vi "rszvl_core_global.vi"() -> ()   [LabVIEW 2014] (continued)
Low,Upp\r\n\nRemote-control command(s):\nCALCulate<1|2>:ATV:LIMit:RESult:CARRiers:<S1PRelative | S2PRelative>:<LOWer | UPPer>?", "Flags"={"OPC Wait"=FALSE, "Dont check status"=FALSE, "*WAI"=FALSE}, "Check Status Callback"=""}, {"Level"=3, "Descriptive Name"="CATV Analog TV Frequency Offset Limit, Vision Carrier Result", "Class Only"=FALSE, "Data Type"=0, "Access"=0, "Identifier"="RSZVL_ATTR_CATV_ATV_CARR_LIM_VCF_RESULT", "Range Table"="rszvl_rngCatvResults", "Command"="CALC:ATV:LIM:RES:CARR:VCF:{ModifLowUpp}?", "Read Callback"="", "Write Callback"="", "Range Callback"="", "Check Callback"="", "Rngtable Callback"="", "Coerce Callback"="", "User Callback"="", "Supported Models"="", "Instrument Options"="", "Repeated Capabilities"="", "Restricted Repeated Capabilities"="", "Help"="This attribute performs a limit check for the frequency offset of the vision carrier.\n\nAvailable Repeated Capabilities:\nModifLowUpp: Low,Upp\r\n\nRemote-control command(s):\nCALCulate<1|2>:ATV:LIMit:RESult:CARRiers:VCFoffset:<LOWer | UPPer>?", "Flags"={"OPC Wait"=FALSE, "Dont check status"=FALSE, "*WAI"=FALSE}, "Check Status Callback"=""}, {"Level"=3, "Descriptive Name"="CATV Analog TV Absolute Limit, Vision Carrier Result", "Class Only"=FALSE, "Data Type"=0, "Access"=0, "Identifier"="RSZVL_ATTR_CATV_ATV_CARR_LIM_VCP_RESULT", "Range Table"="rszvl_rngCatvResults", "Command"="CALC:ATV:LIM:RES:CARR:VCP:{ModifLowUpp}?", "Read Callback"="", "Write Callback"="", "Range Callback"="", "Check Callback"="", "Rngtable Callback"="", "Coerce Callback"="", "User Callback"="", "Supported Models"="", "Instrument Options"="", "Repeated Capabilities"="", "Restricted Repeated Capabilities"="", "Help"="This attribute performs a limit check for the absolute vision carrier power.\n\nAvailable Repeated Capabilities:\nModifLowUpp: Low,Upp\r\n\nRemote-control command(s):\nCALCulate<1|2>:ATV:LIMit:RESult:CARRiers:VCPabsolute:<LOWer | UPPer>?", "Flags"={"OPC Wait"=FALSE, "Dont check status"=FALSE, "*WAI"=FALSE}, "Check Status Callback"=""}, {"Level"=3, "Descriptive Name"="CATV Analog TV Carrier to Noise Ratio Limit Result", "Class Only"=FALSE, "Data Type"=0, "Access"=0, "Identifier"="RSZVL_ATTR_CATV_ATV_LIM_CN_RESULT", "Range Table"="rszvl_rngCatvResults", "Command"="CALC:ATV:LIM:RES:CN:CN:{ModifLowUpp}?", "Read Callback"="", "Write Callback"="", "Range Callback"="", "Check Callback"="", "Rngtable Callback"="", "Coerce Callback"="", "User Callback"="", "Supported Models"="", "Instrument Options"="", "Repeated Capabilities"="", "Restricted Repeated Capabilities"="", "Help"="This attribute performs a limit check for the carrier–to–noise ratio.\n\nNote:\n\n(1) Only Lower Limit is available.\n\nAvailable Repeated Capabilities:\nModifLowUpp: Low,Upp\r\n\nRemote-control command(s):\nCALCulate<1|2>:ATV:LIMit:RESult:CN:CN[:LOWer]?", "Flags"={"OPC Wait"=FALSE, "Dont check status"=FALSE, "*WAI"=FALSE}, "Check Status Callback"=""}, {"Level"=3, "Descriptive Name"="CATV Analog TV Carrier to Second Order Beat Ratio Limit Result", "Class Only"=FALSE, "Data Type"=0, "Access"=0, "Identifier"="RSZVL_ATTR_CATV_ATV_LIM_CSO_RESULT", "Range Table"="rszvl_rngCatvResults", "Command"="CALC:ATV:LIM:RES:CSO:CSO:{ModifLowUpp}?", "Read Callback"="", "Write Callback"="", "Range Callback"="", "Check Callback"="", "Rngtable Callback"="", "Coerce Callback"="", "User Callback"="", "Supported Models"="", "Instrument Options"="", "Repeated Capabilities"="", "Restricted Repeated Capabilities"="", "Help"="This attribute performs a limit check for the carrier–to–second order beat ratio.\n\nNote:\n\n(1) Only Lower Limit is available\n\nAvailable Repeated Capabilities:\nModifLowUpp: Low,Upp\r\n\nRemote-control command(s):\nCALCulate<1|2>:ATV:LIMit:RESult:CSO:CSO[:LOWer]?", "Flags"={"OPC Wait"=FALSE, "Dont check status"=FALSE, "*WAI"=FALSE}, "Check Status Callback"=""}, {"Level"=3, "Descriptive Name"="CATV Analog TV Carrier to Composite Triple Beat Ratio Limit Result", "Class Only"=FALSE, "Data Type"=0, "Access"=0, "Identifier"="RSZVL_ATTR_CATV_ATV_LIM_CTB_RESULT", "Range Table"="rszvl_rngCatvResults", "Command"="CALC:ATV:LIM:RES:CTB:CTB:{ModifLowUpp}?", "Read Callback"="", "Write Callback"="", "Range Callback"="", "Check Callback"="", "Rngtable Callback"="", "Coerce Callback"="", "User Callback"="", "Supported Models"="", "Instrument Options"="", "Repeated Capabilities"="", "Restricted Repeated Capabilities"="", "Help"="This attribute performs a limit check for the carrier–to–composite triple beat ratio.\n\nNote:\n\n(1) Only Lower Limit is available.\n\nAvailable Repeated Capabilities:\nModifLowUpp: Low,Upp\r\n\nRemote-control command(s):\nCALCulate<1|2>:ATV:LIMit:RESult:CTB:CTB[:LOWer]?", "Flags"={"OPC Wait"=FALSE, "Dont check status"=FALSE, "*WAI"=FALSE}, "Check Status Callback"=""}, {"Level"=3, "Descriptive Name"="CATV Analog TV Hum Limit Result", "Class Only"=FALSE, "Data Type"=0, "Access"=0, "Identifier"="RSZVL_ATTR_CATV_ATV_LIM_HUM_RESULT", "Range Table"="rszvl_rngCatvResults", "Command"="CALC:ATV:LIM:RES:HUM:HUM:{ModifLowUpp}?", "Read Callback"="", "Write Callback"="", "Range Callback"="", "Check Callback"="", "Rngtable Callback"="", "Coerce Callback"="", "User Callback"="", "Supported Models"="", "Instrument Options"="", "Repeated Capabilities"="", "Restricted Repeated Capabilities"="", "Help"="This attribute performs a limit check for the Hum measurement.\n\nAvailable Repeated Capabilities:\nModifLowUpp: Low,Upp\r\n\nRemote-control command(s):\nCALCulate<1|2>:ATV:LIMit:RESult:HUM:HUM:<LOWer | UPPer>?", "Flags"={"OPC Wait"=FALSE, "Dont check status"=FALSE, "*WAI"=FALSE}, "Check Status Callback"=""}, {"Level"=3, "Descriptive Name"="CATV Analog TV Vision Modulation Result", "Class Only"=FALSE, "Data Type"=0, "Access"=0, "Identifier"="RSZVL_ATTR_CATV_ATV_LIM_VMOD_MDEP_RESULT", "Range Table"="rszvl_rngCatvResults", "Command"="CALC:ATV:LIM:RES:VMOD:{AtvVisionModulResult}:{ModifLowUpp}?", "Read Callback"="", "Write Callback"="", "Range Callback"="", "Check Callback"="", "Rngtable Callback"="", "Coerce Callback"="", "User Callback"="", "Supported Models"="", "Instrument Options"="", "Repeated Capabilities"="", "Restricted Repeated Capabilities"="", "Help"="This attribute performs a limit check for the  Vision Modulation measurement.\n\nAvailable Repeated Capabilities:\nAtvVisionModulResult: VisCarrPow,ResPicture,Depth\r\nModifLowUpp: Low,Upp\r\n\nRemote-control command(s):\nCALCulate<1|2>:ATV:LIMit:RESult:VMODulation:<MDEPth|RPC|VCP>:<LOWer | UPPer>?", "Flags"={"OPC Wait"=FALSE, "Dont check status"=FALSE, "*WAI"=FALSE}, "Check Status Callback"=""}, {"Level"=2, "Descriptive Name"="ATV Results", "Class Only"=TRUE, "Data Type"=0, "Access"=0, "Identifier"="", "Range Table"="", "Command"="", "Read Callback"="", "Write Callback"="", "Range Callback"="", "Check Callback"="", "Rngtable Callback"="", "Coerce Callback"="", "User Callback"="", "Supported Models"="", "Instrument Options"="", "Repeated Capabilities"="", "Restricted Repeated Capabilities"="", "Help"="Attributes that return ATV measurement results.\n\n(1) CATV Get Analog TV Vision Carrier Power Abs:\nThis attribute reads the vision carrier power absolute value of the Carrier Power measurements.\n\n(2) CATV Get Analog TV Vision Carrier Frequency Offset Value:\nThis attribute reads the vision carrier frequency offset value of the Carrier Power measurements.\n\n(3) CATV Get Analog TV Sound Carrier Power Rel Value:\nThis attribute reads the sound carrier power relative value of the Carrier Power measurements.\n\n(4) CATV Get Analog TV Sound Carrier Intercarrier Frequency Offset Value:\nThis attribute reads the sound carrier intercarrier frequency offset value of the Carrier Power measurements.\n\n(5) CATV Get Analog TV Carrier Result Value:\nThis attribute reads the value of the measurements.\n\nNote:\n\n(1) NRBW is valid only for CN measurement\n\n(6) CATV Get Analog TV CN Carrier to Noise Ratio Value:\nThis attribute reads the carrier–to–noise ratio value of the Carrier–to–Noise Ratio measurements.\n\n(7) CATV Get Analog TV CSO Carrier to Second Order Beat Ratio Value:\nThis attribute reads the carrier–to–second order beat ratio value of the Carrier–to–Second Order Beat Ratio measurements.\n\n(8) CATV Get Analog TV CTB Carrier to Composite Triple Beat Ratio Value:\nThis attribute reads the carrier–to–to–composite triple beat beat ratio value of the Carrier–to–Composite Trip Beat Ratio measurements.\n\n(9) CATV Get Analog TV Hum Value:\nThis attribute reads the measurement values of the Hum measurement.\n\n(10) CATV Get Analog TV Vision Modulation Result Value:\nThis attribute reads the result value of Vision Modulation measurements.", "Flags"={"OPC Wait"=FALSE, "Dont check status"=FALSE, "*WAI"=FALSE}, "Check Status Callback"=""}, {"Level"=3, "Descriptive Name"="CATV Get Analog TV Vision Carrier Power Abs", "Class Only"=FALSE, "Data Type"=1, "Access"=0, "Identifier"="RSZVL_ATTR_CATV_ATV_CARR_VCPA", "Range Table"="", "Command"="CALC:ATV:RES:CARR? VCP", "Read Callback"="", "Write Callback"="", "Range Callback"="", "Check Callback"="", "Rngtable Callback"="", "Coerce Callback"="", "User Callback"="", "Supported Models"="", "Instrument Options"="", "Repeated Capabilities"="", "Restricted Repeated Capabilities"="", "Help"="This attribute reads the vision carrier power absolute value of the Carrier Power measurements.\n\nAvailable Repeated Capabilities:\nNone\n\nRemote-control command(s):\nCALCulate<1|2>:ATV:RESult:CARRiers? VCPabsolute", "Flags"={"OPC Wait"=FALSE, "Dont check status"=FALSE, "*WAI"=FALSE}, "Check Status Callback"=""}, {"Level"=3, "Descriptive Name"="CATV Get Analog TV Vision Carrier Frequency Offset Value", "Class Only"=FALSE, "Data Type"=1, "Access"=0, "Identifier"="RSZVL_ATTR_CATV_ATV_CARR_VCF_VALUE", "Range Table"="", "Command"="CALC:ATV:RES:CARR? VCF", "Read Callback"="", "Write Callback"="", "Range Callback"="", "Check Callback"="", "Rngtable Callback"="", "Coerce Callback"="", "User Callback"="", "Supported Models"="", "Instrument Options"="", "Repeated Capabilities"="", "Restricted Repeated Capabilities"="", "Help"="This attribute reads the vision carrier frequency offset value of the Carrier Power measurements.\n\nAvailable Repeated Capabilities:\nNone\n\nRemote-control command(s):\nCALCulate<1|2>:ATV:RESult:CARRiers? VCFoffset", "Flags"={"OPC Wait"=FALSE, "Dont check status"=FALSE, "*WAI"=FALSE}, "Check Status Callback"=""}, {"Level"=3, "Descriptive Name"="CATV Get Analog TV Sound Carrier Power Rel Value", "Class Only"=FALSE, "Data Type"=1, "Access"=0, "Identifier"="RSZVL_ATTR_CATV_ATV_CARR_REL_POWER_VALUE", "Range Table"="", "Command"="CALC:ATV:RES:CARR? {AtvSoundCarrier}PR", "Read Callback"="", "Write Callback"="", "Range Callback"="", "Check Callback"="", "Rngtable Callback"="", "Coerce Callback"="", "User Callback"="", "Supported Models"="", "Instrument Options"="", "Repeated Capabilities"="", "Restricted Repeated Capabilities"="", "Help"="This attribute reads the sound carrier power relative value of the Carrier Power measurements.\n\nAvailable Repeated Capabilities:\nAtvSoundCarrier: SC1,SC2\r\n\nRemote-control command(s):\nCALCulate<1|2>:ATV:RESult:CARRiers? S1PRelative | S2PRelative", "Flags"={"OPC Wait"=FALSE, "Dont check status"=FALSE, "*WAI"=FALSE}, "Check Status Callback"=""}, {"Level"=3, "Descriptive Name"="CATV Get Analog TV Sound Carrier Intercarrier Frequency Offset Value", "Class Only"=FALSE, "Data Type"=1, "Access"=0, "Identifier"="RSZVL_ATTR_CATV_ATV_CARR_FREQ_OFFSET_VALUE", "Range Table"="", "Command"="CALC:ATV:RES:CARR? {AtvSoundCarrier}IF", "Read Callback"="", "Write Callback"="", "Range Callback"="", "Check Callback"="", "Rngtable Callback"="", "Coerce Callback"="", "User Callback"="", "Supported Models"="", "Instrument Options"="", "Repeated Capabilities"="", "Restricted Repeated Capabilities"="", "Help"="This attribute reads the sound carrier intercarrier frequency offset value of the Carrier Power measurements.\n\nAvailable Repeated Capabilities:\nAtvSoundCarrier: SC1,SC2\r\n\nRemote-control command(s):\nCALCulate<1|2>:ATV:RESult:CARRiers? S1IFoffset | S2IFoffset", "Flags"={"OPC Wait"=FALSE, "Dont check status"=FALSE, "*WAI"=FALSE}, "Check Status Callback"=""}, {"Level"=3, "Descriptive Name"="CATV Get Analog TV Carrier Result Value", "Class Only"=FALSE, "Data Type"=1, "Access"=0, "Identifier"="RSZVL_ATTR_CATV_ATV_VALUE", "Range Table"="", "Command"="CALC:ATV:RES:{AtvCarrier}? {AtvCarrierResult}", "Read Callback"="", "Write Callback"="", "Range Callback"="", "Check Callback"="", "Rngtable Callback"="", "Coerce Callback"="", "User Callback"="", "Supported Models"="", "Instrument Options"="", "Repeated Capabilities"="", "Restricted Repeated Capabilities"="", "Help"="This attribute reads the value of the measurements.\n\nNote:\n\n(1) NRBW is valid only for CN measurement\n\nAvailable Repeated Capabilities:\nAtvCarrier: CN,CSO,CTB\r\nAtvCarrierResult: RefPow,NoiseFloorCorr,FreqRel,CR,NoiseRefBw\r\n\nRemote-control command(s):\nCALCulate<1|2>:ATV:RESult:<CN | CSO | CTB>? RPOWer | NFC | MFR | NRBW", "Flags"={"OPC Wait"=FALSE, "Dont check status"=FALSE, "*WAI"=FALSE}, "Check Status Callback"=""}, {"Level"=3, "Descriptive Name"="CATV Get Analog TV CN Carrier to Noise Ratio Value", "Class Only"=FALSE, "Data Type"=1, "Access"=0, "Identifier"="RSZVL_ATTR_CATV_ATV_CN_CN_VALUE", "Range Table"="", "Command"="CALC:ATV:RES:CN? CN", "Read Callback"="", "Write Callback"="", "Range Callback"="", "Check Callback"="", "Rngtable Callback"="", "Coerce Callback"="", "User Callback"="", "Supported Models"="", "Instrument Options"="", "Repeated Capabilities"="", "Restricted Repeated Capabilities"="", "Help"="This attribute reads the carrier–to–noise ratio value of the Carrier–to–Noise Ratio measurements.\n\nAvailable Repeated Capabilities:\nNone\n\nRemote-control command(s):\nCALCulate<1|2>:ATV:RESult:CN? CN", "Flags"={"OPC Wait"=FALSE, "Dont check status"=FALSE, "*WAI"=FALSE}, "Check Status Callback"=""}, {"Level"=3, "Descriptive Name"="CATV Get Analog TV CSO Carrier to Second Order Beat Ratio Value", "Class Only"=FALSE, "Data Type"=1, "Access"=0, "Identifier"="RSZVL_ATTR_CATV_ATV_CSO_CSO_VALUE", "Range Table"="", "Command"="CALC:ATV:RES:CSO? CSO", "Read Callback"="", "Write Callback"="", "Range Callback"="", "Check Callback"="", "Rngtable Callback"="", "Coerce Callback"="", "User Callback"="", "Supported Models"="", "Instrument Options"="", "Repeated Capabilities"="", "Restricted Repeated Capabilities"="", "Help"="This attribute reads the carrier–to–second order beat ratio value of the Carrier–to–Second Order Beat Ratio measurements.\n\nAvailable Repeated Capabilities:\nNone\n\nRemote-control command(s):\nCALCulate<1|2>:ATV:RESult:CSO? CSO", "Flags"={"OPC Wait"=FALSE, "Dont check status"=FALSE, "*WAI"=FALSE}, "Check Status Callback"=""}, {"Level"=3, "Descriptive Name"="CATV Get Analog TV CTB Carrier to Composite Triple Beat Ratio Value", "Class Only"=FALSE, "Data Type"=1, "Access"=0, "Identifier"="RSZVL_ATTR_CATV_ATV_CTB_CTB_VALUE", "Range Table"="", "Command"="CALC:ATV:RES:CTB? CTB", "Read Callback"="", "Write Callback"="", "Range Callback"="", "Check Callback"="", "Rngtable Callback"="", "Coerce Callback"="", "User Callback"="", "Supported Models"="", "Instrument Options"="", "Repeated Capabilities"="", "Restricted Repeated Capabilities"="", "Help"="This attribute reads the carrier–to–to–composite triple beat beat ratio value of the Carrier–to–Composite Trip Beat Ratio measurements.\n\nAvailable Repeated Capabilities:\nNone\n\nRemote-control command(s):\nCALCulate<1|2>:ATV:RESult:CTB? CTB", "Flags"={"OPC Wait"=FALSE, "Dont check status"=FALSE, "*WAI"=FALSE}, "Check Status Callback"=""}, {"Level"=3, "Descriptive Name"="CATV Get Analog TV Hum Value", "Class Only"=FALSE, "Data Type"=1, "Access"=0, "Identifier"="RSZVL_ATTR_CATV_ATV_HUM_VALUE", "Range Table"="", "Command"="CALC:ATV:RES:HUM?", "Read Callback"="", "Write Callback"="", "Range Callback"="", "Check Callback"="", "Rngtable Callback"="", "Coerce Callback"="", "User Callback"="", "Supported Models"="", "Instrument Options"="", "Repeated Capabilities"="", "Restricted Repeated Capabilities"="", "Help"="This attribute reads the measurement values of the Hum measurement.\n\nAvailable Repeated Capabilities:\nNone\n\nRemote-control command(s):\nCALCulate<1|2>:ATV:RESult:HUM?", "Flags"={"OPC Wait"=FALSE, "Dont check status"=FALSE, "*WAI"=FALSE}, "Check Status Callback"=""}, {"Level"=3, "Descriptive Name"="CATV Get Analog TV Vision Modulation Result Value", "Class Only"=FALSE, "Data Type"=1, "Access"=0, "Identifier"="RSZVL_ATTR_CATV_ATV_VMOD_RESULT_VALUE", "Range Table"="", "Command"="CALC:ATV:RES:VMOD? {AtvVisionModulResult}", "Read Callback"="", "Write Callback"="", "Range Callback"="", "Check Callback"="", "Rngtable Callback"="", "Coerce Callback"="", "User Callback"="", "Supported Models"="", "Instrument Options"="", "Repeated Capabilities"="", "Restricted Repeated Capabilities"="", "Help"="This attribute reads the result value of Vision Modulation measurements.\n\nAvailable Repeated Capabilities:\nAtvVisionModulResult: VisCarrPow,ResPicture,Depth\r\n\nRemote-control command(s):\nCALCulate<1|2>:ATV:RESult:VMODulation? VCPower | RPC | MDEPth", "Flags"={"OPC Wait"=FALSE, "Dont check status"=FALSE, "*WAI"=FALSE}, "Check Status Callback"=""}, {"Level"=2, "Descriptive Name"="DTV Settings", "Class Only"=TRUE, "Data Type"=0, "Access"=0, "Identifier"="", "Range Table"="", "Command"="", "Read Callback"="", "Write Callback"="", "Range Callback"="", "Check Callback"="", "Rngtable Callback"="", "Coerce Callback"="", "User Callback"="", "Supported Models"="", "Instrument Options"="", "Repeated Capabilities"="", "Restricted Repeated Capabilities"="", "Help"="Attributes that configure DTV Settings.\n\n(1) CATV Digital TV Measurement:\nThis attribute defines the digital measurement type.\n\n(2) CATV Digital TV Shoulder Measurement:\nThis attribute activates or deactivates the shoulder measurement in accordance to ETSI TR 101290 standard.\n\n(3) CATV Digital TV Echo Pattern Units:\nThis attribute defines the unit of the Echo Pattern measurement.\n\n(4) CATV Digital TV Echo Pattern Velocity Factor:\nThis attribute defines the velocity of propagation of the signal in the transmission channel (e.g. cable), relative to speed of light.\n\n(5) CATV Digital TV Error Measurements Units:\nThis attribute defines the unit in the Overview / Modulation Errors measurement.\n\n(6) CATV Digital TV Equalizer State:\nThis attribute activates or deactivates the equalizer.\n\n(7) CATV Digital TV Equalizer Freeze:\nThis attribute defines the change of the equalizer coefficients.\n\n(8) CATV Digital TV Equalizer Reset:\nThis attribute resets the equalizer and all equalizer parameters are set to their default values.\n\n(9) CATV Digital TV Roll Off:\nThis attribute defines the roll–off.\n\n(10) CATV Digital TV Symbol Rate:\nThis attribute defines the symbol rate.\n\n(11) CATV Digital TV Standard:\nThis attribute sets the TV standard for Digital TV\n\n(12) CATV Digital TV Constellation Parameter:\nThis attribute sets the constellation parameter for digital TV measurements.", "Flags"={"OPC Wait"=FALSE, "Dont check status"=FALSE, "*WAI"=FALSE}, "Check Status Callback"=""}, {"Level"=3, "Descriptive Name"="CATV Digital TV Measurement", "Class Only"=FALSE, "Data Type"=0, "Access"=2, "Identifier"="RSZVL_ATTR_CATV_DTV_MEAS", "Range Table"="rszvl_rngCatvDtvMeas", "Command"="CONF:DTV:MEAS", "Read Callback"="", "Write Callback"="", "Range Callback"="", "Check Callback"="", "Rngtable Callback"="", "Coerce Callback"="", "User Callback"="", "Supported Models"="", "Instrument Options"="", "Repeated Capabilities"="", "Restricted Repeated Capabilities"="", "Help"="This attribute defines the digital measurement type.\n\nAvailable Repeated Capabilities:\nNone\n\nRemote-control command(s):\nCONFigure:DTV:MEASurement DSPectrum | CHPower | CONS | MERRors | EPATtern | APD | CCDF | OVERview", "Flags"={"OPC Wait"=FALSE, "Dont check status"=FALSE, "*WAI"=FALSE}, "Check Status Callback"=""}, {"Level"=3, "Descriptive Name"="CATV Digital TV Shoulder Measurement", "Class Only"=FALSE, "Data Type"=3, "Access"=2, "Identifier"="RSZVL_ATTR_CATV_DTV_SATT", "Range Table"="", "Command"="CONF:DTV:MEAS:SATT", "Read Callback"="", "Write Callback"="", "Range Callback"="", "Check Callback"="", "Rngtable Callback"="", "Coerce Callback"="", "User Callback"="", "Supported Models"="", "Instrument Options"="", "Repeated Capabilities"="", "Restricted Repeated Capabilities"="", "Help"="This attribute activates or deactivates the shoulder measurement in accordance to ETSI TR 101290 standard.\n\nAvailable Repeated Capabilities:\nNone\n\nRemote-control command(s):\nCONFigure:DTV:MEASurement:SATTenuation ON | OFF", "Flags"={"OPC Wait"=FALSE, "Dont check status"=FALSE, "*WAI"=FALSE}, "Check Status Callback"=""}, {"Level"=3, "Descriptive Name"="CATV Digital TV Echo Pattern Units", "Class Only"=FALSE, "Data Type"=0, "Access"=2, "Identifier"="RSZVL_ATTR_CATV_DTV_EPAT_UNIT", "Range Table"="rszvl_rngUnitSecMin", "Command"="CALC:DTV:UNIT:POW:EPAT", "Read Callback"="", "Write Callback"="", "Range Callback"="", "Check Callback"="", "Rngtable Callback"="", "Coerce Callback"="", "User Callback"="", "Supported Models"="", "Instrument Options"="", "Repeated Capabilities"="", "Restricted Repeated Capabilities"="", "Help"="This attribute defines the unit of the Echo Pattern measurement.\n\nAvailable Repeated Capabilities:\nNone\n\nRemote-control command(s):\nCALCulate<1|2>:DTV:UNIT:POWer:EPATtern", "Flags"={"OPC Wait"=FALSE, "Dont check status"=FALSE, "*WAI"=FALSE}, "Check Status Callback"=""}, {"Level"=3, "Descriptive Name"="CATV Digital TV Echo Pattern Velocity Factor", "Class Only"=FALSE, "Data Type"=1, "Access"=2, "Identifier"="RSZVL_ATTR_CATV_DTV_EPAT_RVEL", "Range Table"="rszvl_rngCatvDtvEPattVelocity", "Command"="CORR:RVEL", "Read Callback"="", "Write Callback"="", "Range Callback"="", "Check Callback"="", "Rngtable Callback"="", "Coerce Callback"="", "User Callback"="", "Supported Models"="", "Instrument Options"="", "Repeated Capabilities"="", "Restricted Repeated Capabilities"="", "Help"="This attribute defines the velocity of propagation of the signal in the transmission channel (e.g. cable), relative to speed of light.\n\nAvailable Repeated Capabilities:\nNone\n\nRemote-control command(s):\n[SENSe<1|2>:]CORRection:RVELocity", "Flags"={"OPC Wait"=FALSE, "Dont check status"=FALSE, "*WAI"=FALSE}, "Check Status Callback"=""}, {"Level"=3, "Descriptive Name"="CATV Digital TV Error Measurements Units", "Class Only"=FALSE, "Data Type"=0, "Access"=2, "Identifier"="RSZVL_ATTR_CATV_DTV_ERROR_UNIT", "Range Table"="rszvl_rngUnitDbPct", "Command"="CALC:DTV:UNIT:POW:{DtvErrorMeas}", "Read Callback"="", "Write Callback"="", "Range Callback"="", "Check Callback"="", "Rngtable Callback"="", "Coerce Callback"="", "User Callback"="", "Supported Models"="", "Instrument Options"="", "Repeated Capabilities"="", "Restricted Repeated Capabilities"="", "Help"="This attribute defines the unit in the Overview / Modulation Errors measurement.\n\nAvailable Repeated Capabilities:\nDtvErrorMeas: EVMPeak,EVMRms,MERPeak,MERRms\r\n\nRemote-control command(s):\nCALCulate<1|2>:DTV:UNIT:POWer:<EVMPeak | EVMRms | MERPeak | MERRms>", "Flags"={"OPC Wait"=FALSE, "Dont check status"=FALSE, "*WAI"=FALSE}, "Check Status Callback"=""}, {"Level"=3, "Descriptive Name"="CATV Digital TV Equalizer State", "Class Only"=FALSE, "Data Type"=3, "Access"=2, "Identifier"="RSZVL_ATTR_CATV_DTV_EQUALIZER_STATE", "Range Table"="", "Command"="DDEM:EQU", "Read Callback"="", "Write Callback"="", "Range Callback"="", "Check Callback"="", "Rngtable Callback"="", "Coerce Callback"="", "User Callback"="", "Supported Models"="", "Instrument Options"="", "Repeated Capabilities"="", "Restricted Repeated Capabilities"="", "Help"="This attribute activates or deactivates the equalizer.\n\nAvailable Repeated Capabilities:\nNone\n\nRemote-control command(s):\n[SENSe<1|2>:]DDEMod:EQUalizer[:STATe]", "Flags"={"OPC Wait"=FALSE, "Dont check status"=FALSE, "*WAI"=FALSE}, "Check Status Callback"=""}, {"Level"=3, "Descriptive Name"="CATV Digital TV Equalizer Freeze", "Class Only"=FALSE, "Data Type"=3, "Access"=2, "Identifier"="RSZVL_ATTR_CATV_DTV_EQUALIZER_FREEZE", "Range Table"="", "Command"="DDEM:EQU:FRE", "Read Callback"="", "Write Callback"="", "Range Callback"="", "Check Callback"="", "Rngtable Callback"="", "Coerce Callback"="", "User Callback"="", "Supported Models"="", "Instrument Options"="", "Repeated Capabilities"="", "Restricted Repeated Capabilities"="", "Help"="This attribute defines the change of the equalizer coefficients.\n\nAvailable Repeated Capabilities:\nNone\n\nRemote-control command(s):\n[SENSe<1|2>:]DDEMod:EQUalizer:FREeze[:STATe]", "Flags"={"OPC Wait"=FALSE, "Dont check status"=FALSE, "*WAI"=FALSE}, "Check Status Callback"=""}, {"Level"=3, "Descriptive Name"="CATV Digital TV Equalizer Reset", "Class Only"=FALSE, "Data Type"=4, "Access"=1, "Identifier"="RSZVL_ATTR_CATV_DTV_EQUALIZER_RESET", "Range Table"="", "Command"="DDEM:EQU:RES", "Read Callback"="", "Write Callback"="", "Range Callback"="", "Check Callback"="", "Rngtable Callback"="", "Coerce Callback"="", "User Callback"="", "Supported Models"="", "Instrument Options"="", "Repeated Capabilities"="", "Restricted Repeated Capabilities"="", "Help"="This attribute resets the equalizer and all equalizer parameters are set to their default values.\n\nAvailable Repeated Capabilities:\nNone\n\nRemote-control command(s):\n[SENSe<1|2>:]DDEMod:EQUalizer:RESet", "Flags"={"OPC Wait"=FALSE, "Dont check status"=FALSE, "*WAI"=FALSE}, "Check Status Callback"=""}, {"Level"=3, "Descriptive Name"="CATV Digital TV Roll Off", "Class Only"=FALSE, "Data Type"=0, "Access"=2, "Identifier"="RSZVL_ATTR_CATV_DTV_FILTER_ALPHA", "Range Table"="rszvl_rngCatvDtvFilterAlpha", "Command"="DDEM:FILT:ALPH", "Read Callback"="", "Write Callback"="", "Range Callback"="", "Check Callback"="", "Rngtable Callback"="", "Coerce Callback"="", "User Callback"="", "Supported Models"="", "Instrument Options"="", "Repeated Capabilities"="", "Restricted Repeated Capabilities"="", "Help"="This attribute defines the roll–off.\n\nAvailable Repeated Capabilities:\nNone\n\nRemote-control command(s):\n[SENSe<1|2>:]DDEMod:FILTer:ALPHa", "Flags"={"OPC Wait"=FALSE, "Dont check status"=FALSE, "*WAI"=FALSE}, "Check Status Callback"=""}, {"Level"=3, "Descriptive Name"="CATV Digital TV Symbol Rate", "Class Only"=FALSE, "Data Type"=1, "Access"=2, "Identifier"="RSZVL_ATTR_CATV_DTV_SRATE", "Range Table"="", "Command"="DDEM:SRAT", "Read Callback"="", "Write Callback"="", "Range Callback"="", "Check Callback"="", "Rngtable Callback"="", "Coerce Callback"="", "User Callback"="", "Supported Models"="", "Instrument Options"="", "Repeated Capabilities"="", "Restricted Repeated Capabilities"="", "Help"="This attribute defines the symbol rate.\n\nAvailable Repeated Capabilities:\nNone\n\nRemote-control command(s):\n[SENSe<1|2>:]DDEMod:SRATe", "Flags"={"OPC Wait"=FALSE, "Dont check status"=FALSE, "*WAI"=FALSE}, "Check Status Callback"=""}, {"Level"=3, "Descriptive Name"="CATV Digital TV Standard", "Class Only"=FALSE, "Data Type"=0, "Access"=2, "Identifier"="RSZVL_ATTR_CATV_DTV_STANDARD", "Range Table"="rszvl_rngCatvDtvStandard", "Command"="SET:TV:STAN", "Read Callback"="", "Write Callback"="", "Range Callback"="", "Check Callback"="", "Rngtable Callback"="", "Coerce Callback"="", "User Callback"="", "Supported Models"="", "Instrument Options"="", "Repeated Capabilities"="", "Restricted Repeated Capabilities"="", "Help"="This attribute sets the TV standard for Digital TV\n\nAvailable Repeated Capabilities:\nNone\n\nRemote-control command(s):\nSETup:TV:STANdard J83A | J83B | J83C", "Flags"={"OPC Wait"=FALSE, "Dont check status"=FALSE, "*WAI"=FALSE}, "Check Status Callback"=""}, {"Level"=3, "Descriptive Name"="CATV Digital TV Constellation Parameter", "Class Only"=FALSE, "Data Type"=0, "Access"=2, "Identifier"="RSZVL_ATTR_CATV_DTV_FORMAT", "Range Table"="rszvl_rngCatvDtvFormat", "Command"="SOUR:DM:FORM", "Read Callback"="", "Write Callback"="", "Range Callback"="", "Check Callback"="", "Rngtable Callback"="", "Coerce Callback"="", "User Callback"="", "Supported Models"="", "Instrument Options"="", "Repeated Capabilities"="", "Restricted Repeated Capabilities"="", "Help"="This attribute sets the constellation parameter for digital TV measurements.\n\nAvailable Repeated Capabilities:\nNone\n\nRemote-control command(s):\nSOURce:DM:FORMat QAM4 | QAM16 | QAM32 | QAM64 | QAM128 | QAM256 | QAM512 | QAM1024", "Flags"={"OPC Wait"=FALSE, "Dont check status"=FALSE, "*WAI"=FALSE}, "Check Status Callback"=""}, {"Level"=2, "Descriptive Name"="DTV Limit Settings", "Class Only"=TRUE, "Data Type"=0, "Access"=0, "Identifier"="", "Range Table"="", "Command"="", "Read Callback"="", "Write Callback"="", "Range Callback"="", "Check Callback"="", "Rngtable Callback"="", "Coerce Callback"="", "User Callback"="", "Supported Models"="", "Instrument Options"="", "Repeated Capabilities"="", "Restricted Repeated Capabilities"="", "Help"="Attributes that configure DTV Limit Settings.\n\n(1) CATV Digital TV Carrier Frequency Offset Limit:\nThis attribute defines the limit of the carrier frequency offset in the Overview measurement.\n\n(2) CATV Digital TV Channel Power Limit:\nThis attribute defines the limit for the Channel Power measurement.\n\n(3) CATV Digital TV Carrier Suppression Limit:\nThis attribute defines the limit of the carrier suppression in the Modulation Errors measurement.\n\nNote:\n\n(1) Only Lower Limit is available\n\n(4) CATV Digital TV Error Limit Lower:\nThis attribute defines the lower limit of the Overview/Modulation Errors measurement.\n\n(5) CATV Digital TV Error Limit Upper:\nThis attribute defines the upper limit of the  Overview/Modulation Errors measurement.\n\n(6) CATV Digital TV IQ Imbalance Limit:\nThis attribute defines the limit of the I/Q amplitude imbalance value in the Modulation Errors measurement.\n\n(7) CATV Digital TV Phase Jitter Limit:\nThis attribute defines the upper limit of the phase jitter (root mean square value of the phase error) in the Modulation Errors measurement.\n\nNote:\n\n(1) Only Upper Limit is availlable\n\n(8) CATV Digital TV Quadrature Error Limit:\nThis attribute defines the limit of the quadrature error in the Modulation Errors measurement.\n\n(9) CATV Digital TV Symbol Rate Offset Limit:\nThis attribute defines the limit of the symbol rate offset in the Overview measurement.", "Flags"={"OPC Wait"=FALSE, "Dont check status"=FALSE, "*WAI"=FALSE}, "Check Status Callback"=""}, {"Level"=3, "Descriptive Name"="CATV Digital TV Carrier Frequency Offset Limit", "Class Only"=FALSE, "Data Type"=1, "Access"=2, "Identifier"="RSZVL_ATTR_CATV_DTV_CARR_LIM_FREQ_OFFSET", "Range Table"="rszvl_rngCatvFreqOffset", "Command"="CALC:DTV:LIM:CFOF:{ModifLowUpp}", "Read Callback"="", "Write Callback"="", "Range Callback"="", "Check Callback"="", "Rngtable Callback"="", "Coerce Callback"="", "User Callback"="", "Supported Models"="", "Instrument Options"="", "Repeated Capabilities"="", "Restricted Repeated Capabilities"="", "Help"="This attribute defines the limit of the carrier frequency offset in the Overview measurement.\n\nAvailable Repeated Capabilities:\nModifLowUpp: Low,Upp\r\n\nRemote-control command(s):\nCALCulate:DTV:LIMit:CFOFfset:<LOWer | UPPer>", "Flags"={"OPC Wait"=FALSE, "Dont check status"=FALSE, "*WAI"=FALSE}, "Check Status Callback"=""}, {"Level"=3, "Descriptive Name"="CATV Digital TV Channel Power Limit", "Class Only"=FALSE, "Data Type"=1, "Access"=2, "Identifier"="RSZVL_ATTR_CATV_DTV_LIM_CHANNEL_POWER", "Range Table"="rszvl_rngCatvAbsPower", "Command"="CALC:DTV:LIM:CHP:{ModifLowUpp}", "Read Callback"="", "Write Callback"="", "Range Callback"="", "Check Callback"="", "Rngtable Callback"="", "Coerce Callback"="", "User Callback"="", "Supported Models"="", "Instrument Options"="", "Repeated Capabilities"="", "Restricted Repeated Capabilities"="", "Help"="This attribute defines the limit for the Channel Power measurement.\n\nAvailable Repeated Capabilities:\nModifLowUpp: Low,Upp\r\n\nRemote-control command(s):\nCALCulate:DTV:LIMit:CHPower:<LOWer | UPPer>", "Flags"={"OPC Wait"=FALSE, "Dont check status"=FALSE, "*WAI"=FALSE}, "Check Status Callback"=""}, {"Level"=3, "Descriptive Name"="CATV Digital TV Carrier Suppression Limit", "Class Only"=FALSE, "Data Type"=1, "Access"=2, "Identifier"="RSZVL_ATTR_CATV_DTV_LIM_SUPP", "Range Table"="rszvl_rngCatvCarrSuppression", "Command"="CALC:DTV:LIM:CSUP:{ModifLowUpp}", "Read Callback"="", "Write Callback"="", "Range Callback"="", "Check Callback"="", "Rngtable Callback"="", "Coerce Callback"="", "User Callback"="", "Supported Models"="", "Instrument Options"="", "Repeated Capabilities"="", "Restricted Repeated Capabilities"="", "Help"="This attribute defines the limit of the carrier suppression in the Modulation Errors measurement.\n\nNote:\n\n(1) Only Lower Limit is available\n\nAvailable Repeated Capabilities:\nModifLowUpp: Low,Upp\r\n\nRemote-control command(s):\nCALCulate:DTV:LIMit:CSUPpression[:LOWer]", "Flags"={"OPC Wait"=FALSE, "Dont check status"=FALSE, "*WAI"=FALSE}, "Check Status Callback"=""}, {"Level"=3, "Descriptive Name"="CATV Digital TV Error Limit Lower", "Class Only"=FALSE, "Data Type"=1, "Access"=2, "Identifier"="RSZVL_ATTR_CATV_DTV_LIM_ERR_LOW", "Range Table"="rszvl_rngCatvErrLimitLower", "Command"="CALC:DTV:LIM:{DtvErrorMeas}:LOW", "Read Callback"="", "Write Callback"="", "Range Callback"="", "Check Callback"="", "Rngtable Callback"="", "Coerce Callback"="", "User Callback"="", "Supported Models"="", "Instrument Options"="", "Repeated Capabilities"="", "Restricted Repeated Capabilities"="", "Help"="This attribute defines the lower limit of the Overview/Modulation Errors measurement.\n\nAvailable Repeated Capabilities:\nDtvErrorMeas: EVMPeak,EVMRms,MERPeak,MERRms\r\n\nRemote-control command(s):\nCALCulate:DTV:LIMit:<EVMPeak | EVMRms | MERPeak | MERRms>:LOWer", "Flags"={"OPC Wait"=FALSE, "Dont check status"=FALSE, "*WAI"=FALSE}, "Check Status Callback"=""}, {"Level"=3, "Descriptive Name"="CATV Digital TV Error Limit Upper", "Class Only"=FALSE, "Data Type"=1, "Access"=2, "Identifier"="RSZVL_ATTR_CATV_DTV_LIM_ERR_UPP", "Range Table"="rszvl_rngCatvErrLimitUpper", "Command"="CALC:DTV:LIM:{DtvErrorMeas}:UPP", "Read Callback"="", "Write Callback"="", "Range Callback"="", "Check Callback"="", "Rngtable Callback"="", "Coerce Callback"="", "User Callback"="", "Supported Models"="", "Instrument Options"="", "Repeated Capabilities"="", "Restricted Repeated Capabilities"="", "Help"="This attribute defines the upper limit of the  Overview/Modulation Errors measurement.\n\nAvailable Repeated Capabilities:\nDtvErrorMeas: EVMPeak,EVMRms,MERPeak,MERRms\r\n\nRemote-control command(s):\nCALCulate:DTV:LIMit:<EVMPeak | EVMRms | MERPeak | MERRms>:UPPer", "Flags"={"OPC Wait"=FALSE, "Dont check status"=FALSE, "*WAI"=FALSE}, "Check Status Callback"=""}, {"Level"=3, "Descriptive Name"="CATV Digital TV IQ Imbalance Limit", "Class Only"=FALSE, "Data Type"=1, "Access"=2, "Identifier"="RSZVL_ATTR_CATV_DTV_LIM_IMB", "Range Table"="rszvl_rngCatvImbLimit", "Command"="CALC:DTV:LIM:IMB:{ModifLowUpp}", "Read Callback"="", "Write Callback"="", "Range Callback"="", "Check Callback"="", "Rngtable Callback"="", "Coerce Callback"="", "User Callback"="", "Supported Models"="", "Instrument Options"="", "Repeated Capabilities"="", "Restricted Repeated Capabilities"="", "Help"="This attribute defines the limit of the I/Q amplitude imbalance value in the Modulation Errors measurement.\n\nAvailable Repeated Capabilities:\nModifLowUpp: Low,Upp\r\n\nRemote-control command(s):\nCALCulate:DTV:LIMit:IMBalance:<LOWer | UPPer>", "Flags"={"OPC Wait"=FALSE, "Dont check status"=FALSE, "*WAI"=FALSE}, "Check Status Callback"=""}, {"Level"=3, "Descriptive Name"="CATV Digital TV Phase Jitter Limit", "Class Only"=FALSE, "Data Type"=1, "Access"=2, "Identifier"="RSZVL_ATTR_CATV_DTV_LIM_PJIT", "Range Table"="rszvl_rngCatvPhaseJitterLimit", "Command"="CALC:DTV:LIM:PJIT:{ModifLowUpp}", "Read Callback"="", "Write Callback"="", "Range Callback"="", "Check Callback"="", "Rngtable Callback"="", "Coerce Callback"="", "User Callback"="", "Supported Models"="", "Instrument Options"="", "Repeated Capabilities"="", "Restricted Repeated Capabilities"="", "Help"="This attribute defines the upper limit of the phase jitter (root mean square value of the phase error) in the Modulation Errors measurement.\n\nNote:\n\n(1) Only Upper Limit is availlable\n\nAvailable Repeated Capabilities:\nModifLowUpp: Low,Upp\r\n\nRemote-control command(s):\nCALCulate:DTV:LIMit:PJITter[:UPPer]", "Flags"={"OPC Wait"=FALSE, "Dont check status"=FALSE, "*WAI"=FALSE}, "Check Status Callback"=""}, {"Level"=3, "Descriptive Name"="CATV Digital TV Quadrature Error Limit", "Class Only"=FALSE, "Data Type"=1, "Access"=2, "Identifier"="RSZVL_ATTR_CATV_DTV_LIM_QERR", "Range Table"="rszvl_rngCatvQuadratureErrLimit", "Command"="CALC:DTV:LIM:QERR:{ModifLowUpp}", "Read Callback"="", "Write Callback"="", "Range Callback"="", "Check Callback"="", "Rngtable Callback"="", "Coerce Callback"="", "User Callback"="", "Supported Models"="", "Instrument Options"="", "Repeated Capabilities"="", "Restricted Repeated Capabilities"="", "Help"="This attribute defines the limit of the quadrature error in the Modulation Errors measurement.\n\nAvailable Repeated Capabilities:\nModifLowUpp: Low,Upp\r\n\nRemote-control command(s):\nCALCulate:DTV:LIMit:QERRor:<LOWer | UPPer>", "Flags"={"OPC Wait"=FALSE, "Dont check status"=FALSE, "*WAI"=FALSE}, "Check Status Callback"=""}, {"Level"=3, "Descriptive Name"="CATV Digital TV Symbol Rate Offset Limit", "Class Only"=FALSE, "Data Type"=1, "Access"=2, "Identifier"="RSZVL_ATTR_CATV_DTV_LIM_SYMB_RATE_OFFSET", "Range Table"="rszvl_rngCatvSymbRateLimit", "Command"="CALC:DTV:LIM:SROF:{ModifLowUpp}", "Read Callback"="", "Write Callback"="", "Range Callback"="", "Check Callback"="", "Rngtable Callback"="", "Coerce Callback"="", "User Callback"="", "Supported Models"="", "Instrument Options"="", "Repeated Capabilities"="", "Restricted Repeated Capabilities"="", "Help"="This attribute defines the limit of the symbol rate offset in the Overview measurement.\n\nAvailable Repeated Capabilities:\nModifLowUpp: Low,Upp\r\n\nRemote-control command(s):\nCALCulate:DTV:LIMit:SROFfset:<LOWer | UPPer>", "Flags"={"OPC Wait"=FALSE, "Dont check status"=FALSE, "*WAI"=FALSE}, "Check Status Callback"=""}, {"Level"=2, "Descriptive Name"="DTV Limit Results", "Class Only"=TRUE, "Data Type"=0, "Access"=0, "Identifier"="", "Range Table"="", "Command"="", "Read Callback"="", "Write Callback"="", "Range Callback"="", "Check Callback"="", "Rngtable Callback"="", "Coerce Callback"="", "User Callback"="", "Supported Models"="", "Instrument Options"="", "Repeated Capabilities"="", "Restricted Repeated Capabilities"="", "Help"="Attributes that return DTV limit results.\n\n(1) CATV Digital TV Carrier Frequency Offset Limit Result:\nThis attribute performs a limit check for the carrier frequency offset in the Overview measurement.\n\n(2) CATV Digital TV Channel Power Limit Result:\nThis attribute queries the result of the Channel Power measurement. Upper and lower limit check can not be handled separately.\n\n(3) CATV Digital TV Carrier Suppression Limit Result:\nThis attribute performs a limit check for the lower limit of the carrier suppression in the Modulation Errors measurement. \n\n(4) CATV Digital TV Error Limit Result:\nThis attribute performs an limit check for the Overview/Modulation Errors measurement.\n\n(5) CATV Digital TV IQ Imbalance Limit Result:\nThis attribute performs a limit check for the I/Q amplitude imbalance value in the Modulation Errors measurement.\n\n(6) CATV Digital TV Phase Jitter Limit Result:\nThis attribute performs an limit check for the phase jitter in the Modulation Errors measurement.\n
